vi "Fire Stop.vi"(8 "error in (no error)":errorcluster) -> (0 "error out":errorcluster)   [LabVIEW 2018]
uses:
  Controles/FGV Opciones.ctl
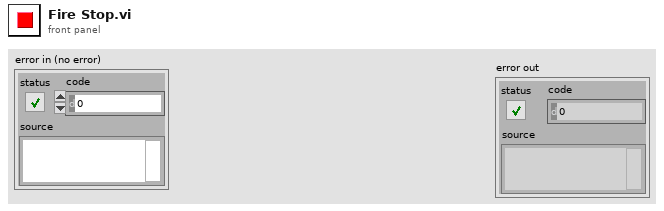
[diagram p1: front panel]
types:
  T1 = typedef "FGV Opciones.ctl" = enum16{"Get", "Create", "Destroy"}
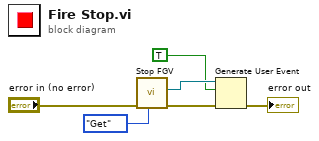
[diagram p0: block diagram]
diagram:
  n1 = call "Stop FGV.vi"("Enum"=FGV_Opciones."Get", "error in (no error)"="error in (no error)") -> ("error out"=w6:errorcluster, "Stop"=w4:refnum<user-event>)  [unwired: 7 in, 1 out]
  n2 = Generate User Event(user event=w4, event data cluster=TRUE ("event data"), error in=w6) -> (error out=→"error out":errorcluster)  [unwired: 1 in, 1 out]
